vi "FlexRIO_CPUDAQ.vi"() -> ()   [LabVIEW 2013]
uses:
  <vilib>/rvi/Emulation/niFpgaSctlEmulationGetInTimedLoop.vi
  <vilib>/rvi/Emulation/niFpgaEmulationReportErrorSimple.vi
  <vilib>/rvi/Emulation/niFpgaGetClockAttributes.vi
  <vilib>/rvi/interface/RandomDataEmulation/nirviRandomDataFPGAFIFO.vi
  <vilib>/rvi/interface/RandomDataEmulation/niFpgaRandomDataHandleErrors.vi
  <vilib>/rvi/Emulation/niFpgaCriticalErrorInLSC.vi
  <vilib>/rvi/DataTransferAndStorage/Container/XNode/niFpgaContainer.xnode
  <vilib>/rvi/interface/RandomDataEmulation/nirviRandomDataFpgaReadWriteTemplate.vi
panel:
  out "DMATtoHOSTBlockNWords":u16[](array[numeric])
  out "SGFref1":u32=100000000
  in  "SGSignalType1":u8
  in  "SGUpdateRate1":u32=40
  in  "SGPhase1":u32
  in  "SGFreq1":u32=100000
  in  "SGAmp1":u16
  out "SGFref0":u32=100000000
  in  "SGSignalType0":u8
  in  "SGUpdateRate0":u32=40
  in  "SGPhase0":u32
  in  "SGFreq0":u32=100000
  in  "SGAmp0":u16
  out "SGNo":u8=2
  out "PXIIN1":bool
  in  "PXIOUT1":bool
  out "PXIIN0":bool
  in  "PXIOUT0":bool
  out "auxDI1":bool
  out "auxDI0":bool
  out "DI1":bool
  out "DI0":bool
  in  "auxDO1":bool
  in  "auxDO0":bool
  in  "DO1":bool
  in  "DO0":bool
  in  "AOEnable1":bool
  in  "AOEnable0":bool
  in  "auxAO1":i32
  in  "auxAO0":i32
  in  "AO1":i32
  in  "AO0":i32
  out "auxAI1":i32
  out "auxAI0":i32
  out "AI1":i32
  out "AI0":i32
  in  "DMATtoHOSTEnable1":bool
  in  "DMATtoHOSTSamplingRate1":u16=10000
  out "DMATtoHOSTOverflows":u16
  in  "DMATtoHOSTSamplingRate0":u16=10000
  in  "DMATtoHOSTEnable0":bool
  out "DMATtoHOSTSampleSize":u8[](array[numeric])
  out "DMATtoHOSTFrameType":u8[](array[numeric])
  out "DMATtoHOSTNCh":u16[](array[numeric])
  out "Platform":enum8{"FlexRIO", "cRIO", "RSeries"}(ring)
  in  "DebugMode":bool
  in  "DAQStartStop":bool
  out "DevProfile":T1(ring)
  out "DevTemp":i16=-10244
  out "DevQualityStatus":u8
  out "Fref":u32=100000000
  out "RIOAdapterCorrect":bool=TRUE
  out "InsertedIOModule ID":u32
  out "InitDone":bool=TRUE
  out "FPGAVIversion":u8[](array[numeric])=[1, 0]
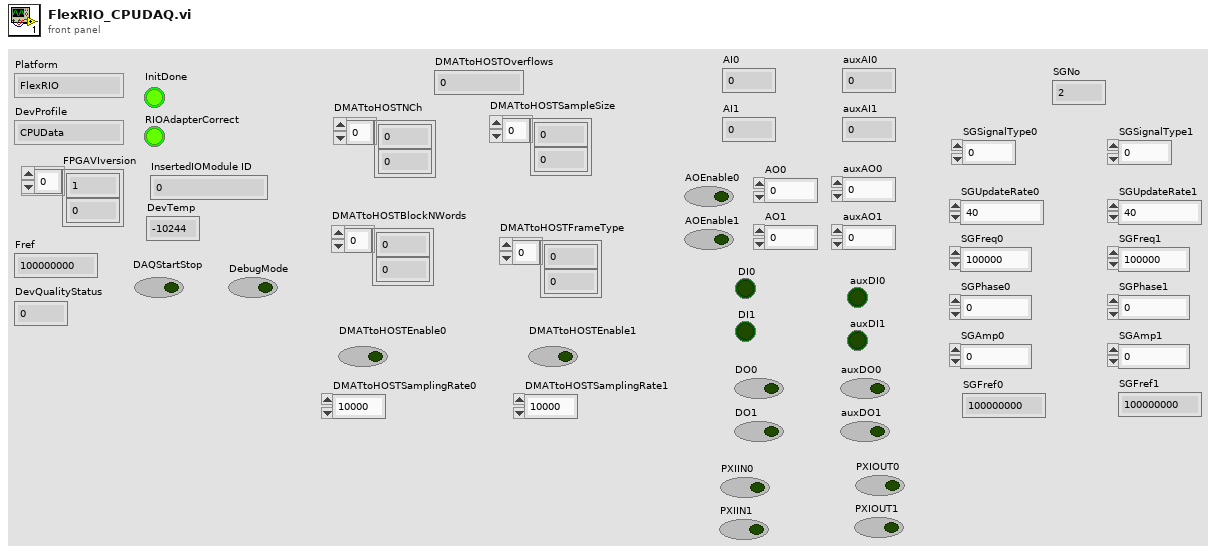
[diagram p1: front panel]
types:
  T1 = enum8{"CPUData", "CPUImage", "GPUData", "GPUImage"}
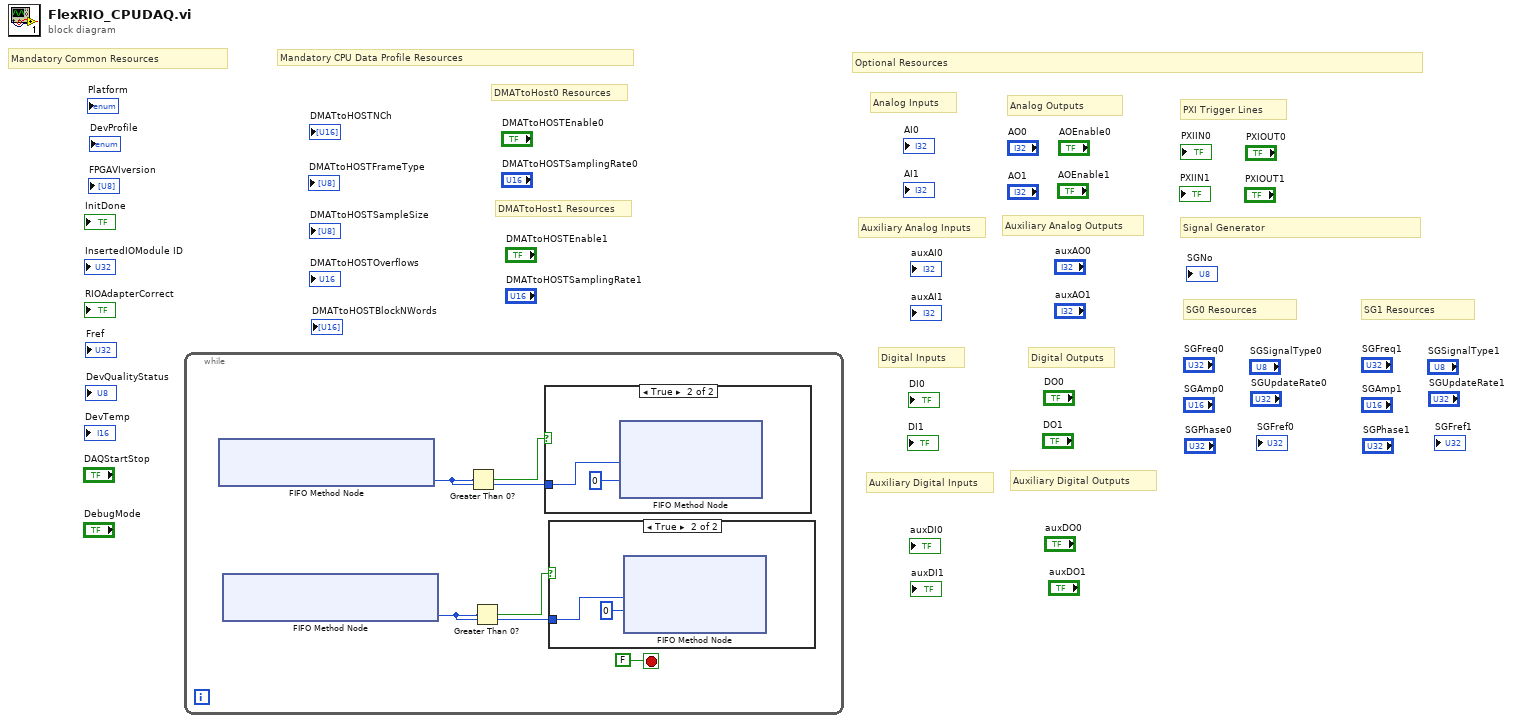
[diagram p0: block diagram]
diagram:
  # "SG1 Resources"
  # "SG0 Resources"
  # "Signal Generator"
  # "PXI Trigger Lines"
  # "Digital Outputs"
  # "Auxiliary Digital Outputs"
  # "Auxiliary Digital Inputs"
  # "Digital Inputs"
  # "Auxiliary Analog Outputs"
  # "Analog Outputs"
  # "Auxiliary Analog Inputs"
  # "Analog Inputs"
  # "Optional Resources"
  # "DMATtoHost1 Resources"
  # "DMATtoHost0 Resources"
  # "Mandatory CPU Data Profile Resources"
  # "Mandatory Common Resources"
  n1 = while {
    stop <- FALSE stop-if-true
    n2 = xnode ("FIFO Method Node")() -> ("Number of Elements to Write"=w3:u32)  [unwired: 1 in, 1 out]
    n3 = xnode ("FIFO Method Node")() -> ("Number of Elements to Write"=w2:u32)  [unwired: 1 in, 1 out]
    n4 = Greater Than 0?(x=w3) -> (x > 0?=w4:bool)
    n5 = Greater Than 0?(x=w2) -> (x > 0?=w1:bool)
    n6 = case shown="True" w4 {
      tunnel: w3 -> [_ w9]
      frame False {
      }
      frame True {
        n7 = xnode ("FIFO Method Node")("Element"=w9, "Timeout"=i16 0) -> ()  [unwired: 1 in, 2 out]
      }
    }
    n8 = case shown="True" w1 {
      tunnel: w2 -> [_ w7]
      frame False {
      }
      frame True {
        n9 = xnode ("FIFO Method Node")("Element"=w7, "Timeout"=i16 0) -> ()  [unwired: 1 in, 2 out]
      }
    }
  }
